vi "SubVI - Receive Config File.vi"(11 "file path (use dialog)":path) -> (0 "error out":errorcluster)   [LabVIEW 2017]
panel:
  out "Array":string[][](array[string])
  out "Progress ( % )":u8
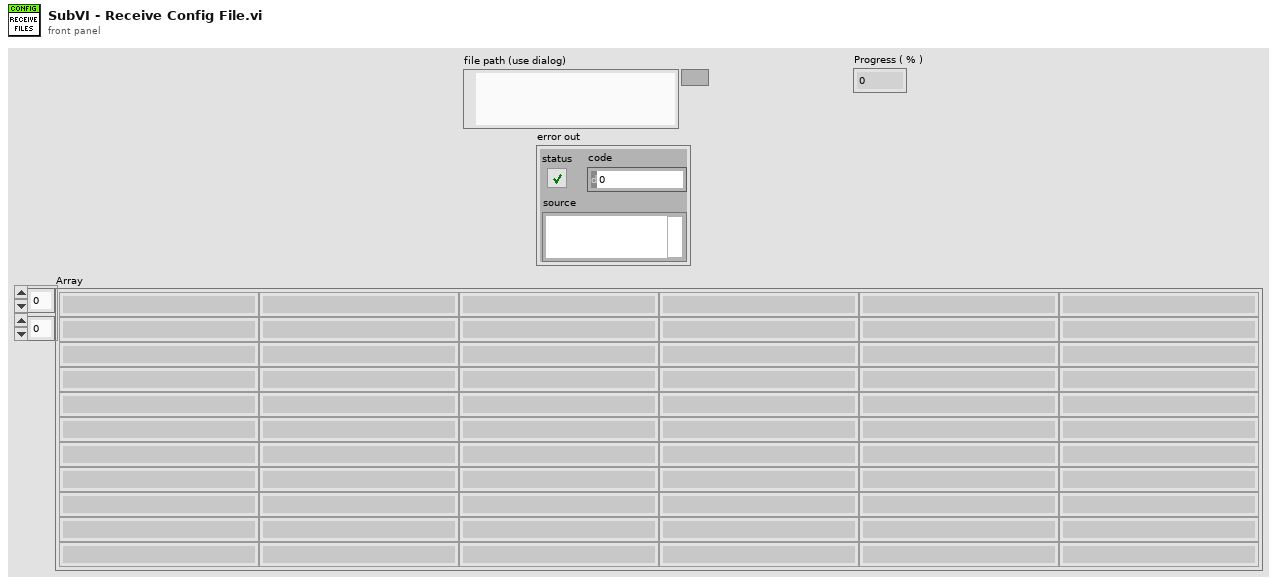
[diagram p1: front panel]
types:
  T1 = enum16{"open", "replace", "create", "open or create", "replace or create", "replace or create with confirmation"}
  T2 = enum16{"big-endian, network order", "native, host order", "little-endian"}
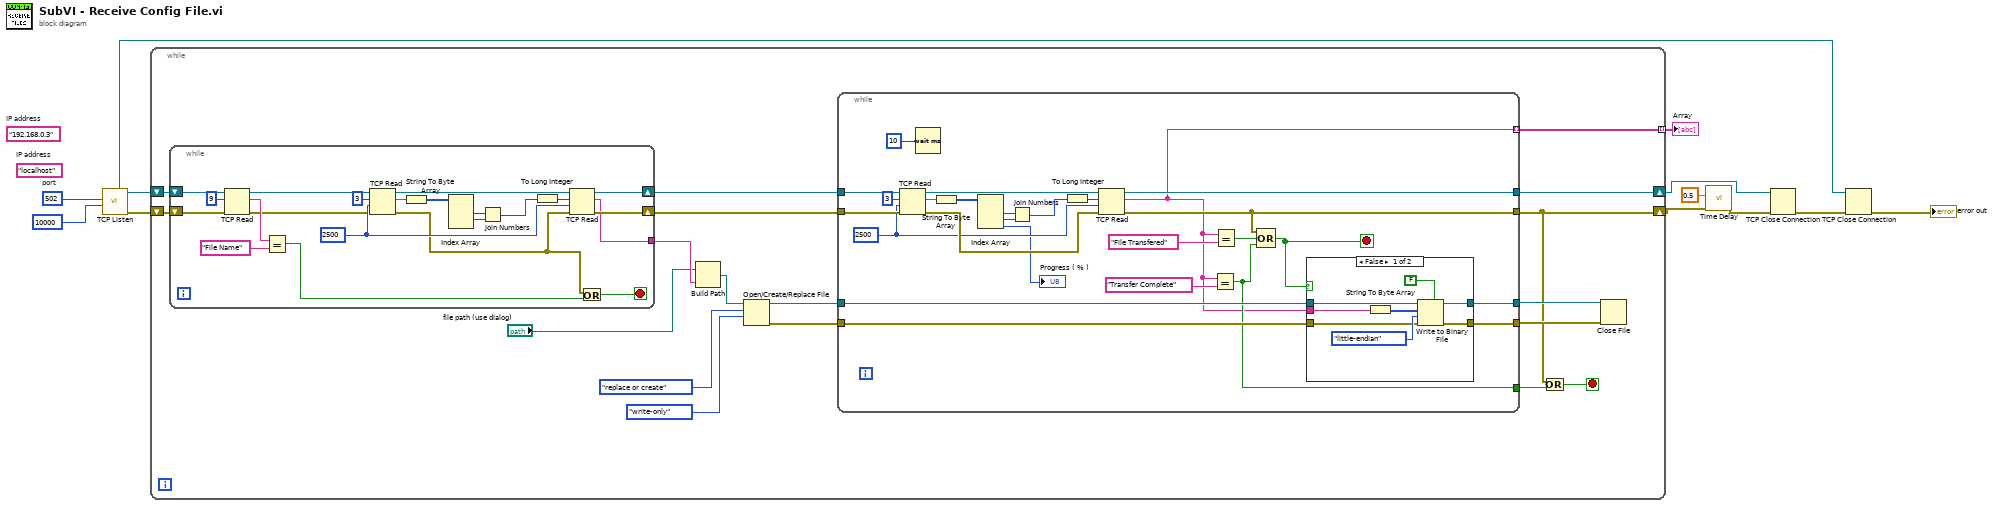
[diagram p0: block diagram]
diagram:
  (unwired) "192.168.0.3"  # IP address
  w12 = u16 502  # port
  (unwired) "localhost"  # IP address
  n1 = call <vilib>:"TCP Listen.vi"("timeout ms (wait forever: -1)"=10000, "port"=w12) -> ("error out"=w9:errorcluster, "connection ID"=w10:refnum<k5>, "listener ID"=w3:refnum<k5>)  [unwired: 5 in, 2 out]
  n2 = while {
    shift-right: [w17] -> w8
    shift-left: w10 -> [w24]
    shift-right: [w14] -> w7
    shift-left: w9 -> [w26]
    tunnel: [w13] -> w4 mode=indexing
    stop <- w15 stop-if-true
    n3 = while {
      shift-right: [w35] -> w25
      shift-left: w26 -> [w49]
      shift-right: [w36] -> w23
      shift-left: w24 -> [w48]
      tunnel: [w33] -> w22
      stop <- w32 stop-if-true
      w39 = 2500 ("timeout ms (25000)")
      n4 = TCP Read(connection ID=w48, bytes to read=9, error in (no error)=w49) -> (connection ID out=w38:refnum<k5>, data out=w51:string, error out=w37:errorcluster)  [unwired: 2 in]
      n5 = Equal?(x=w51, y="File Name" ("data in")) -> (x = y?=w34:bool)
      n6 = TCP Read(connection ID=w38, bytes to read=3, error in (no error)=w37, 9:w39) -> (connection ID out=w42:refnum<k5>, data out=w46:string, error out=w31:errorcluster)  [unwired: 1 in]
      n7 = String To Byte Array(string=w46) -> (unsigned byte array=w45:u8[])
      n8 = Index Array(array=w45) -> (element #1=w44:u8, element #2=w43:u8)  [unwired: 3 in, 1 out]
      n9 = Join Numbers(hi=w44, lo=w43) -> ((hi.lo)=w40:u16)
      n10 = To Long Integer(number=w40) -> (32bit integer=w41:i32)
      n11 = TCP Read(connection ID=w42, bytes to read=w41, error in (no error)=w31, 9:w39) -> (connection ID out=w36:refnum<k5>, data out=w33:string, error out=w35:errorcluster)  [unwired: 1 in]
      n12 = Or(x=w31, y=w34) -> (x .or. y?=w32:bool)
    }
    n13 = Build Path(base path="file path (use dialog)", name or relative path=w22) -> (appended path=w20:path)
    n14 = Open/Create/Replace File(file path (use dialog)=w20, operation (0:open)=T1."replace or create", access (0:read/write)=enum16{"read/write", "read-only", "write-only"}."write-only") -> (refnum out=w27:refnum<file>, error out=w28:errorcluster)  [unwired: 3 in, 1 out]
    n15 = while {
      tunnel: w23 -> [w78]
      tunnel: w25 -> [w77]
      tunnel: [w68] -> w17
      tunnel: [w54] -> w14
      tunnel: w28 -> [w66]
      tunnel: w27 -> [w65]
      tunnel: [w64] -> w18
      tunnel: [w63] -> w19
      tunnel: [w55] -> w16
      tunnel: [w53] -> w13 mode=indexing
      stop <- w56 stop-if-true
      w60 = 2500 ("timeout ms (25000)")
      n16 = TCP Read(connection ID=w78, bytes to read=3, error in (no error)=w77, 9:w60) -> (connection ID out=w71:refnum<k5>, data out=w75:string, error out=w70:errorcluster)  [unwired: 1 in]
      n17 = Wait (ms)(milliseconds to wait=u32 10) -> ()  [unwired: 1 out]
      n18 = String To Byte Array(string=w75) -> (unsigned byte array=w74:u8[])
      n19 = Index Array(array=w74) -> (element #1=w73:u8, element #2=w72:u8, element #3=→"Progress ( % )":u8)  [unwired: 3 in]
      n20 = Join Numbers(hi=w73, lo=w72) -> ((hi.lo)=w61:u16)
      n21 = To Long Integer(number=w61) -> (32bit integer=w69:i32)
      n22 = TCP Read(connection ID=w71, bytes to read=w69, error in (no error)=w70, 9:w60) -> (connection ID out=w68:refnum<k5>, data out=w53:string, error out=w54:errorcluster)  [unwired: 1 in]
      n23 = Equal?(x=w53, y="Transfer Complete" ("data in")) -> (x = y?=w55:bool)
      n24 = Equal?(x=w53, y="File Transfered" ("data in")) -> (x = y?=w62:bool)
      n25 = Compound Arithmetic op=OR(w54, w62, w55) -> (w56:bool)
      n26 = case shown="False" w56 {
        tunnel: w66 -> [w84 w87]
        tunnel: w65 -> [w83 w88]
        tunnel: [w82 w88] -> w64
        tunnel: [w81 w87] -> w63
        tunnel: w53 -> [w80 _]
        frame False {
          n27 = String To Byte Array(string=w80) -> (unsigned byte array=w79:u8[])
          n28 = Write to Binary File(file (use dialog)=w83, data=w79, error in=w84, 5:FALSE ("prepend array or string size? (T)"), 9:T2."little-endian" ("byte order (0:big-endian, network order)")) -> (refnum out=w82:refnum<file>, error out=w81:errorcluster)  [unwired: 1 in, 1 out]
        }
        frame True {
        }
      }
    }
    n29 = Or(x=w14, y=w16) -> (x .or. y?=w15:bool)
    n30 = Close File(refnum=w18, error in=w19) -> ()  [unwired: 2 out]
  }
  "Array" <- w4
  n31 = call "Time Delay"("error in (no error)"=w7, "Delay Time (s)"=0.5) -> ("error out"=w6:errorcluster)  [unwired: 9 in]
  n32 = TCP Close Connection(connection ID=w8, error in (no error)=w6) -> (error out=w2:errorcluster)  [unwired: 1 in, 1 out]
  n33 = TCP Close Connection(connection ID=w3, error in (no error)=w2) -> (error out=→"error out":errorcluster)  [unwired: 1 in, 1 out]
